vi "Field List Parse Values.vi"(10 "nDataType":T1, 11 "sValue":string) -> (2 "js List Array":string, 3 "Current Value":string)   [LabVIEW 2011]
uses:
  Field DataTypes.ctl
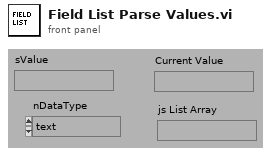
[diagram p1: front panel]
types:
  T1 = typedef "Field DataTypes.ctl" = enum32{"text", "numeric", "list", "timestamp", "boolean"}
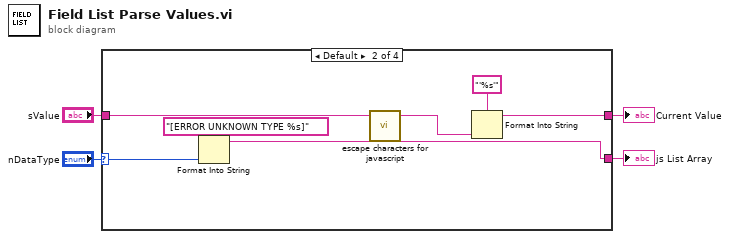
[diagram p0: block diagram]
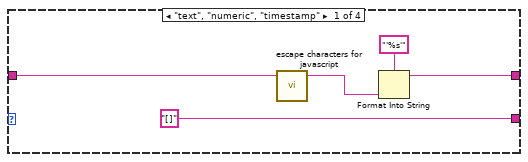
[diagram p2: hidden frame]
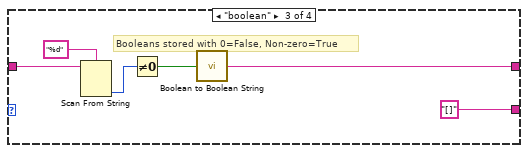
[diagram p3: hidden frame]
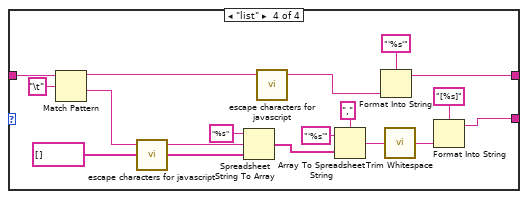
[diagram p4: hidden frame]
diagram:
  n1 = case shown="Default" "nDataType" {
    selector: "nDataType" -> [_ w12 _ _]
    tunnel: "sValue" -> [w8 w16 w21 w37]
    tunnel: [w5 w13 w17 w24] -> w2
    tunnel: ["[]" w10 "[]" w38] -> w1
    frame "text", "numeric", "timestamp" {
      n2 = call "escape characters for javascript.vi"("String (\"\")"=w8) -> ("escaped String"=w6:string)  [unwired: 4 out]
      n3 = Format Into String(format string="'%s'", w6) -> (resulting string=w5:string)  [unwired: 2 in, 1 out]
    }
    frame Default {
      n4 = Format Into String(format string="[ERROR UNKNOWN TYPE %s]", w12) -> (resulting string=w10:string)  [unwired: 2 in, 1 out]
      n5 = call "escape characters for javascript.vi"("String (\"\")"=w16) -> ("escaped String"=w14:string)  [unwired: 4 out]
      n6 = Format Into String(format string="'%s'", w14) -> (resulting string=w13:string)  [unwired: 2 in, 1 out]
    }
    frame "boolean" {
      # "Booleans stored with 0=False, Non-zero=True"
      n7 = Scan From String(format string="%d", input string=w21) -> (output 1=w19:i32)  [unwired: 2 in, 4 out]
      n8 = Not Equal To 0?(x=w19) -> (x != 0?=w18:bool)
      n9 = call "Boolean to Boolean String.vi"("Boolean"=w18) -> ("Boolean string"=w17:string)  [unwired: 1 in]
    }
    frame "list" {
      n10 = Match Pattern(string=w37, regular expression="\t") -> (before substring=w29:string, after substring=w27:string)  [unwired: 3 out]
      n11 = call "escape characters for javascript.vi"("String (\"\")"=w27) -> ("escaped String"=w28:string)  [unwired: 4 out]
      n12 = Spreadsheet String To Array(format string="%s", spreadsheet string=w28, array type (2D Dbl)=string[] []) -> (array=w32:string[])  [unwired: 1 out]
      n13 = call "escape characters for javascript.vi"("String (\"\")"=w29) -> ("escaped String"=w25:string)  [unwired: 4 out]
      n14 = Array To Spreadsheet String(delimiter (Tab)=",", array=w32, 3:"'%s'" ("format string")) -> (spreadsheet string=w31:string)
      n15 = Format Into String(format string="'%s'", w25) -> (resulting string=w24:string)  [unwired: 2 in, 1 out]
      n16 = call <vilib>:"Trim Whitespace.vi"("string"=w31) -> ("trimmed string"=w30:string)  [unwired: 1 in]
      n17 = Format Into String(format string="[%s]", w30) -> (resulting string=w38:string)  [unwired: 2 in, 1 out]
    }
  }
  "js List Array" <- w1
  "Current Value" <- w2
